vi "GUI - SET -  Actor_Name.vi"(8 "error in (no error)":errorcluster, 10 "Actor_Name":string, 11 "Child_1_Class in":refnum<class "GUI_Class.lvclass">) -> (0 "error out":errorcluster, 3 "Child_1_Class out":refnum<class "GUI_Class.lvclass">)   [LabVIEW 2023, in "GUI_Actor.lvlib" / "GUI_Class.lvclass"]
uses:
  GUI_Class.lvclass
  GUI_Class.lvclass/GUI_Class.ctl
  <vilib>/Utility/error.llb/Trim Whitespace One-Sided.vi
panel:
  out "Actor Name Out":string
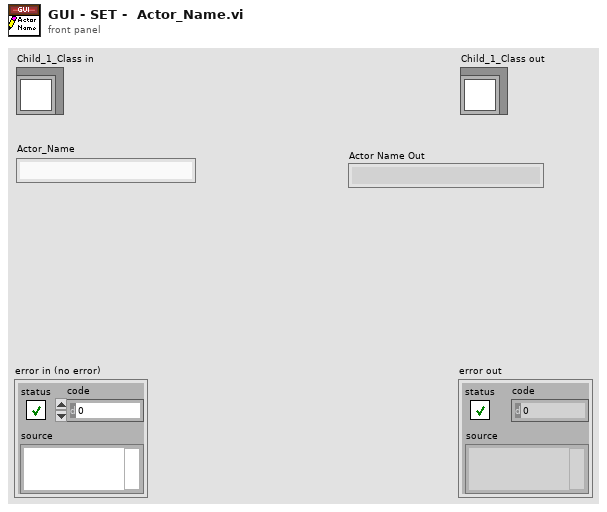
[diagram p1: front panel]
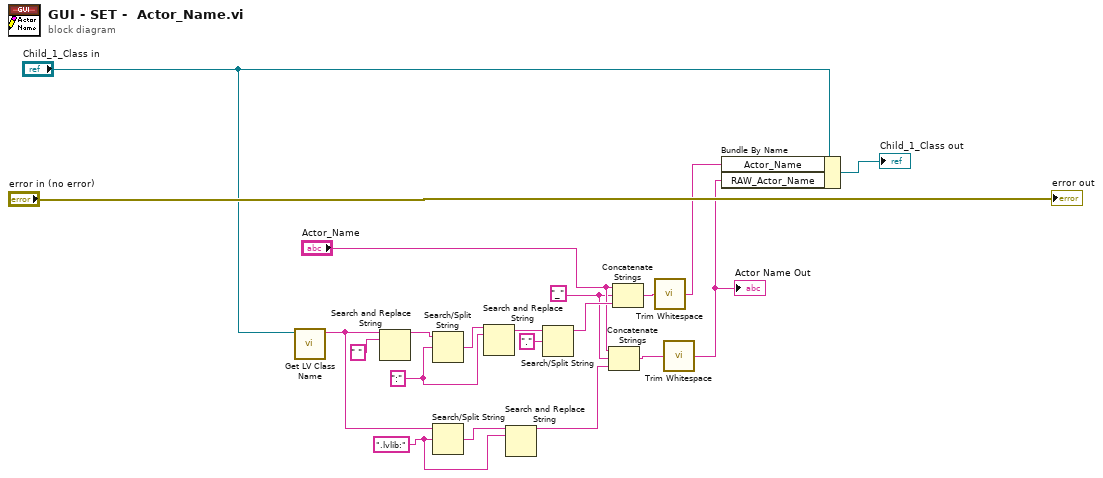
[diagram p0: block diagram]
diagram:
  w7 = ".lvlib:" ("search string/char (-)")
  w15 = ":" ("search string/char (-)")
  w4 = "_" ("string")
  n1 = call <vilib>:"Get LV Class Name.vi"("object"="Child_1_Class in") -> ("class name"=w8:string)  [unwired: 9 in, 1 out]
  n2 = Search and Replace String(input string=w8, search string=" ") -> (result string=w17:string)  [unwired: 6 in, 3 out]
  n3 = Search/Split String(string=w17, search string/char (-)=w15) -> (match + rest of string=w16:string)  [unwired: 1 in, 2 out]
  n4 = Search/Split String(string=w8, search string/char (-)=w7) -> (match + rest of string=w6:string)  [unwired: 1 in, 2 out]
  n5 = Search and Replace String(input string=w16, search string=w15) -> (result string=w13:string)  [unwired: 6 in, 3 out]
  n6 = Search and Replace String(input string=w6, search string=w7) -> (result string=w3:string)  [unwired: 6 in, 3 out]
  n7 = Search/Split String(string=w13, search string/char (-)=".") -> (substring before match=w11:string)  [unwired: 1 in, 2 out]
  n8 = Concatenate Strings("Actor_Name", w4, w3) -> (w2:string)
  n9 = Concatenate Strings("Actor_Name", w4, w11) -> (w14:string)
  n10 = call <vilib>:"Trim Whitespace.vi"("string"=w14) -> ("trimmed string"=w9:string)  [unwired: 1 in]
  n11 = call <vilib>:"Trim Whitespace.vi"("string"=w2) -> ("trimmed string"=w1:string)  [unwired: 1 in]
  "Actor Name Out" <- w1
  n12 = Bundle By Name(cluster="Child_1_Class in", "Actor_Name"=w9, "RAW_Actor_Name"=w1) -> (→"Child_1_Class out":refnum<class "GUI_Class.lvclass">)
  "error out" <- "error in (no error)"
